vi "ReadData2Ch.vi"(0 "object in":refnum<class "AD2_MSO_SDK.lvclass">, 5 "error in (no error)":errorcluster) -> (14 "object out":refnum<class "AD2_MSO_SDK.lvclass">, 16 "Ch1":waveform(dbl), 17 "CH2":waveform(dbl), 19 "error out":errorcluster)   [LabVIEW 2019, in "AD2_MSO_SDK.lvclass"]
uses:
  AD2_MSO_SDK.lvclass
  AD2_MSO_SDK.lvclass/AD2_MSO_SDK.ctl
  Olasdwf/Olasdwf.lvlib
panel:
  out "String":string
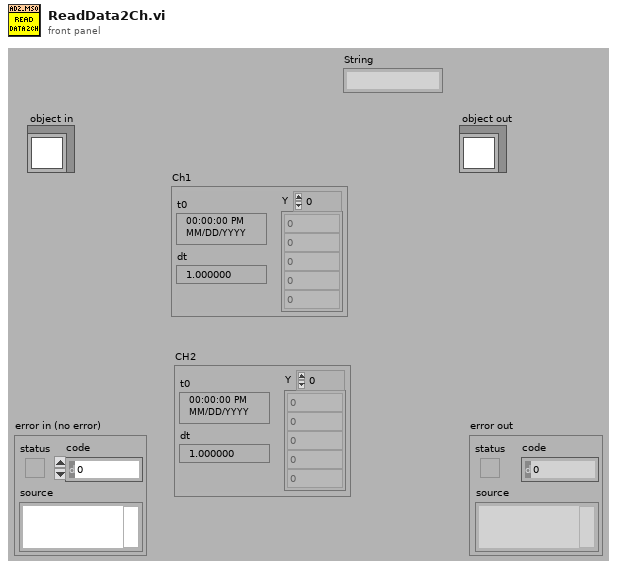
[diagram p1: front panel]
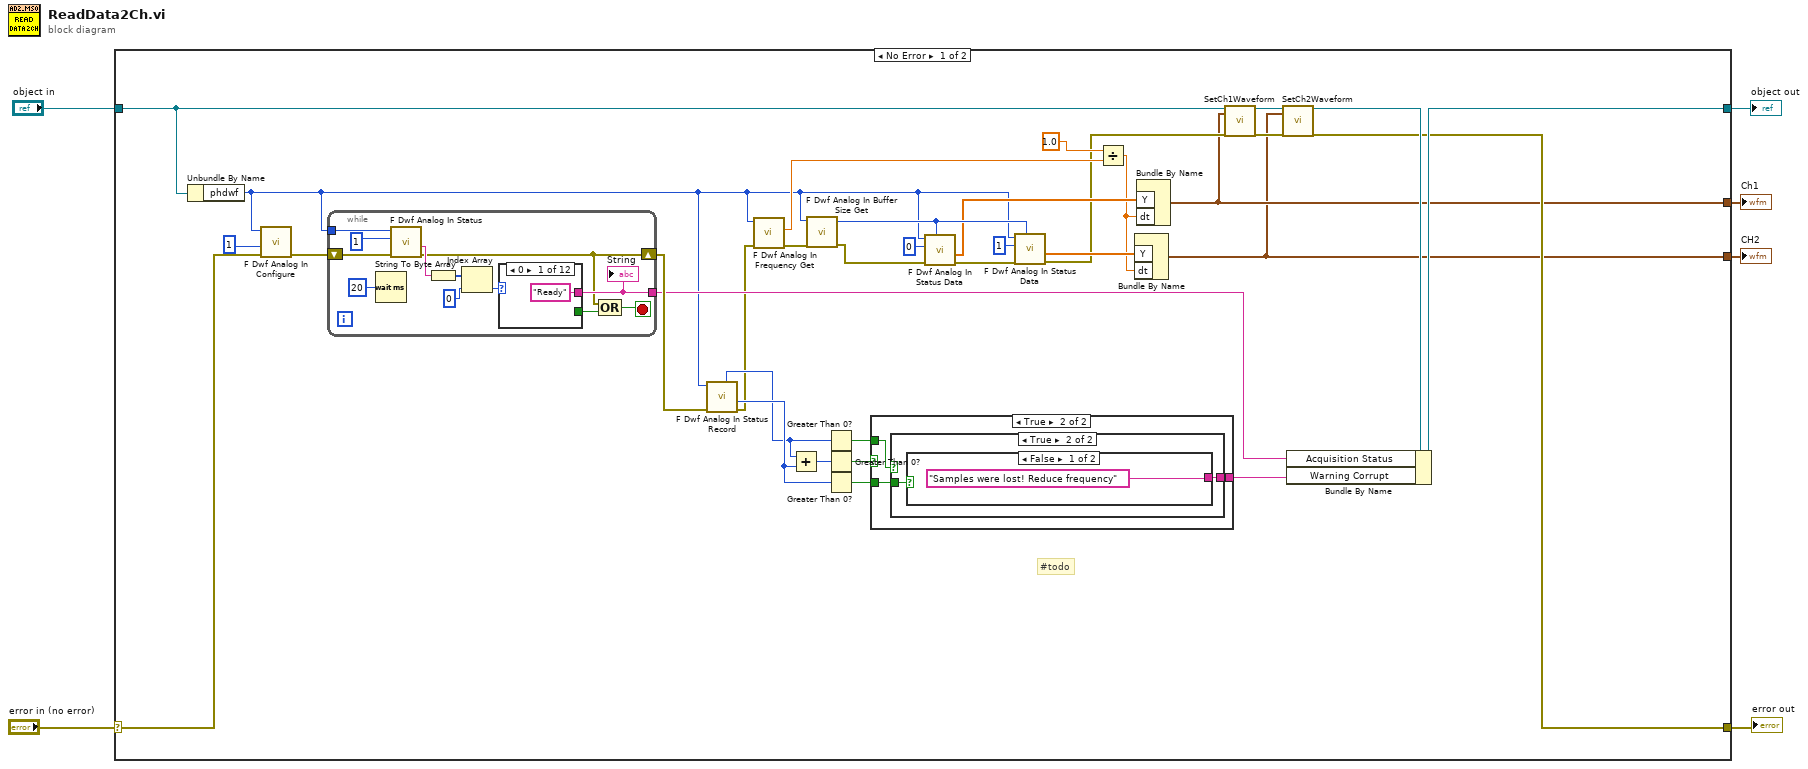
[diagram p0: block diagram]
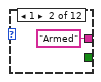
[diagram p2: hidden frame]
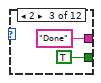
[diagram p3: hidden frame]
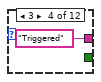
[diagram p4: hidden frame]
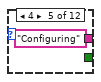
[diagram p5: hidden frame]
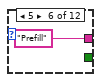
[diagram p6: hidden frame]
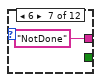
[diagram p7: hidden frame]
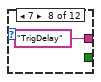
[diagram p8: hidden frame]
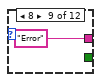
[diagram p9: hidden frame]
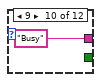
[diagram p10: hidden frame]
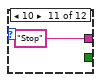
[diagram p11: hidden frame]
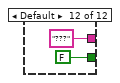
[diagram p12: hidden frame]
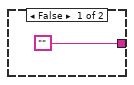
[diagram p13: hidden frame]
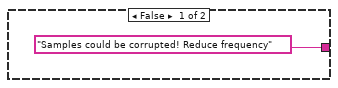
[diagram p14: hidden frame]
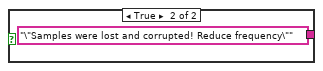
[diagram p15: hidden frame]
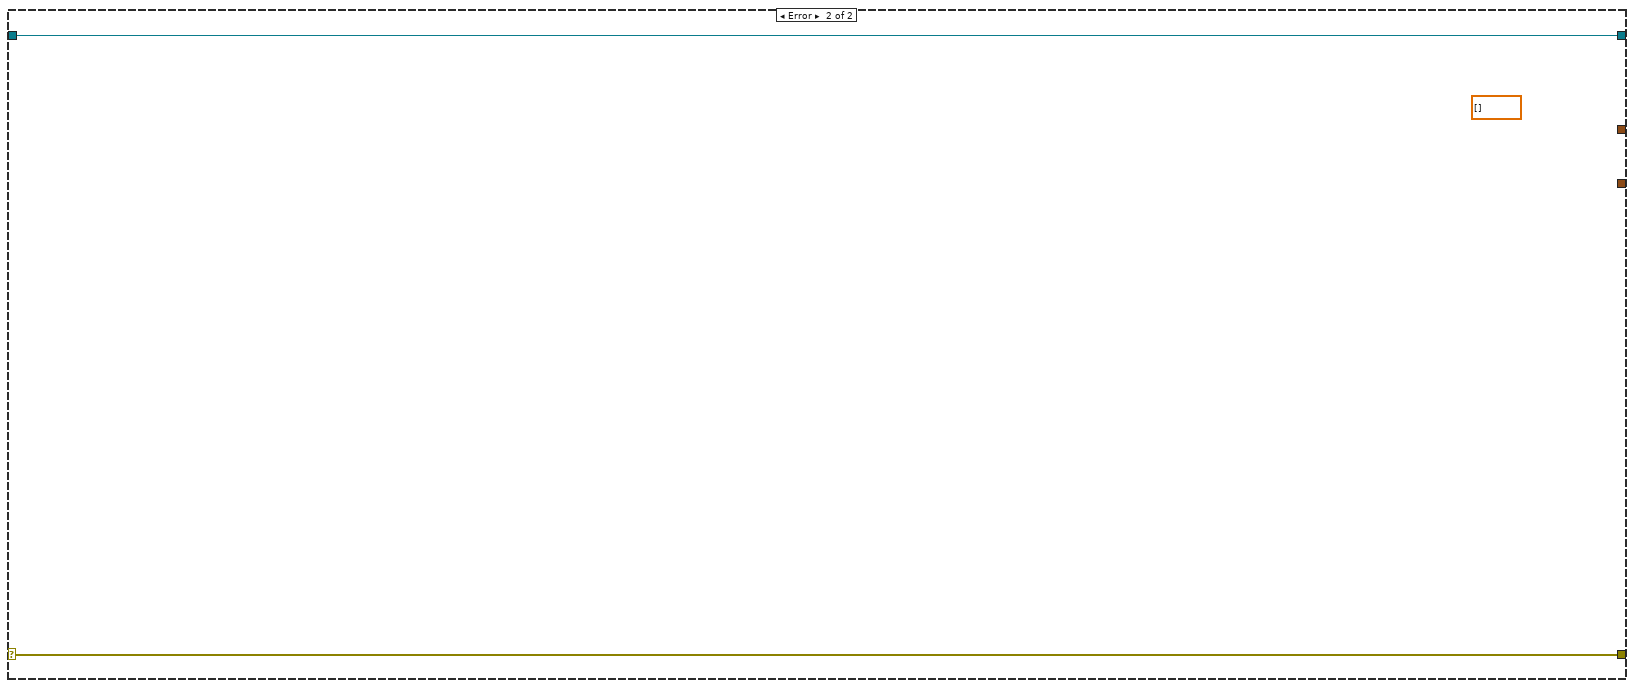
[diagram p16: hidden frame]
diagram:
  n1 = case shown="No Error" "error in (no error)" {
    selector: "error in (no error)" -> [w11 w77]
    tunnel: [w12 w77] -> w5
    tunnel: [w30 w76] -> w3
    tunnel: "object in" -> [w16 w76]
    tunnel: [w8 _] -> w2
    tunnel: [w7 _] -> w1
    frame No Error {
      # "#todo"
      n2 = Unbundle By Name(w16) -> ("phdwf"=w9:i32)
      n3 = call "F Dwf Analog In Configure.vi"("error in (no error)"=w11, "fStart"=1, "hdwf"=w9) -> ("error out"=w10:errorcluster)  [unwired: 7 in, 1 out]
      n4 = while {
        tunnel: [w49] -> w29
        shift-right: [w44] -> w31
        shift-left: w10 -> [w41]
        tunnel: w9 -> [w43]
        stop <- w47 stop-if-true
        n5 = Wait (ms)(milliseconds to wait=u32 20) -> ()  [unwired: 1 out]
        n6 = call "F Dwf Analog In Status.vi"("error in (no error)"=w41, "fReadData"=1, "hdwf"=w43) -> ("error out"=w44:errorcluster, "psts out"=w45:string)  [unwired: 6 in, 1 out]
        n7 = String To Byte Array(string=w45) -> (unsigned byte array=w51:u8[])
        n8 = Index Array(array=w51, index=0) -> (element=w52:u8)
        n9 = case shown="0" w52 {
          tunnel: ["Ready" "Armed" "Done" "Triggered" "Configuring" "Prefill" "NotDone" "TrigDelay" "Error" "Busy" "Stop" "???"] -> w49
          tunnel: [_ _ TRUE _ _ _ _ _ _ _ _ FALSE] -> w46
          frame 0 {
          }
          frame 1 {
          }
          frame 2 {
          }
          frame 3 {
          }
          frame 4 {
          }
          frame 5 {
          }
          frame 6 {
          }
          frame 7 {
          }
          frame 8 {
          }
          frame 9 {
          }
          frame 10 {
          }
          frame Default {
          }
        }
        "String" <- w49
        n10 = Compound Arithmetic op=OR(w44, w46) -> (w47:bool)
      }
      n11 = call "F Dwf Analog In Status Record.vi"("error in (no error)"=w31, "hdwf"=w9) -> ("error out"=w20:errorcluster, "pcdDataLost out"=w36:i32, "pcdDataCorrupt out"=w35:i32)  [unwired: 5 in, 2 out]
      n12 = call "F Dwf Analog In Frequency Get.vi"("error in (no error)"=w20, "hdwf"=w9) -> ("error out"=w21:errorcluster, "phzFrequency out"=w24:dbl)  [unwired: 7 in, 1 out]
      n13 = Add(x=w35, y=w36) -> (x+y=w37:i32)
      n14 = call "F Dwf Analog In Buffer Size Get.vi"("error in (no error)"=w21, "hdwf"=w9) -> ("error out"=w19:errorcluster, "pnSize out"=w27:i32)  [unwired: 7 in, 1 out]
      n15 = Greater Than 0?(x=w35) -> (x > 0?=w38:bool)
      n16 = Greater Than 0?(x=w37) -> (x > 0?=w40:bool)
      n17 = Greater Than 0?(x=w36) -> (x > 0?=w39:bool)
      n18 = case shown="True" w40 {
        tunnel: ["" w70] -> w28
        tunnel: w39 -> [_ w69]
        tunnel: w38 -> [_ w68]
        frame False {
        }
        frame True {
          n19 = case shown="True" w68 {
            tunnel: ["Samples could be corrupted! Reduce frequency" w73] -> w70
            tunnel: w69 -> [_ w72]
            frame False {
            }
            frame True {
              n20 = case shown="False" w72 {
                tunnel: ["Samples were lost! Reduce frequency" "\"Samples were lost and corrupted! Reduce frequency\""] -> w73
                frame False {
                }
                frame True {
                }
              }
            }
          }
        }
      }
      n21 = call "F Dwf Analog In Status Data.vi"("cdData"=w27, "error in (no error)"=w19, "idxChannel"=0, "hdwf"=w9) -> ("error out"=w32:errorcluster, "rgdVoltData"=w25:dbl[])  [unwired: 5 in, 1 out]
      n22 = call "F Dwf Analog In Status Data.vi"("cdData"=w27, "error in (no error)"=w32, "idxChannel"=1, "hdwf"=w9) -> ("error out"=w13:errorcluster, "rgdVoltData"=w22:dbl[])  [unwired: 5 in, 1 out]
      n23 = Divide(x=1.0, y=w24) -> (x/y=w14:dbl)
      n24 = Bundle By Name("Y"=w22, "dt"=w14) -> (w7:waveform(dbl))  [unwired: 1 in]
      n25 = Bundle By Name("Y"=w25, "dt"=w14) -> (w8:waveform(dbl))  [unwired: 1 in]
      n26 = call-dynamic "SetCh1Waveform.vi"("object in"=w16, "Ch1 waveform"=w8, "error in (no error)"=w13) -> ("object out"=w18:refnum<class "AD2_MSO_SDK.lvclass">, "error out"=w15:errorcluster)  [unwired: 15 in]
      n27 = call-dynamic "SetCh2Waveform.vi"("object in"=w18, "Ch2 waveform"=w7, "error in (no error)"=w15) -> ("object out"=w17:refnum<class "AD2_MSO_SDK.lvclass">, "error out"=w12:errorcluster)  [unwired: 15 in]
      n28 = Bundle By Name(cluster=w17, "Acquisition Status"=w29, "Warning Corrupt"=w28) -> (w30:refnum<class "AD2_MSO_SDK.lvclass">)
    }
    frame Error {
      (unwired) dbl[] [] ("rgdVoltData")
    }
  }
  "error out" <- w5
  "object out" <- w3
  "Ch1" <- w2
  "CH2" <- w1
